vi "rename tag in mappings helper.vi"(8 "new tag name":string, 9 "input channel?":bool, 10 "old tag name":string, 11 "Mappings":T1[](array[typedef])) -> (3 "Mappings out":T1[](array[typedef]))   [LabVIEW 2013, in "engine configuration.lvclass"]
uses:
  engine configuration.lvclass
  <vilib>/NI/Tag Bus/table/mapping specification.ctl
  <vilib>/NI/Tag Bus/tag/Data Type.ctl
  <vilib>/NI/Tag Bus/table/mapping.ctl
  <vilib>/NI/Tag Bus/tag/tag descriptor.lvclass
  <vilib>/NI/Tag Bus/table/data table.lvlib
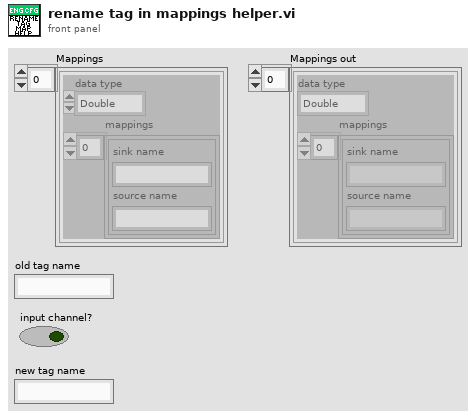
[diagram p1: front panel]
types:
  T1 = typedef "tag bus.lvlib/data table.lvlib/mapping specification.ctl" = cluster{"data type":T2, "mappings":T3[]}
  T2 = typedef "tag bus.lvlib/tag descriptor.lvclass/Data Type.ctl" = enum16{"Double", "Single", "I64", "I32", "I16", "I8", "U64", "U32", "U16", "U8", "Boolean", "String", "Array of Double", "Array of Single", "Array of I64", "Array of I32", "Array of I16", "Array of I8", "Array of U64", "Array of U32", "Array of U16", "Array of U8", "Array of Boolean", "Array of String"}
  T3 = typedef "tag bus.lvlib/data table.lvlib/mapping.ctl" = cluster{"sink name":string, "source name":string}
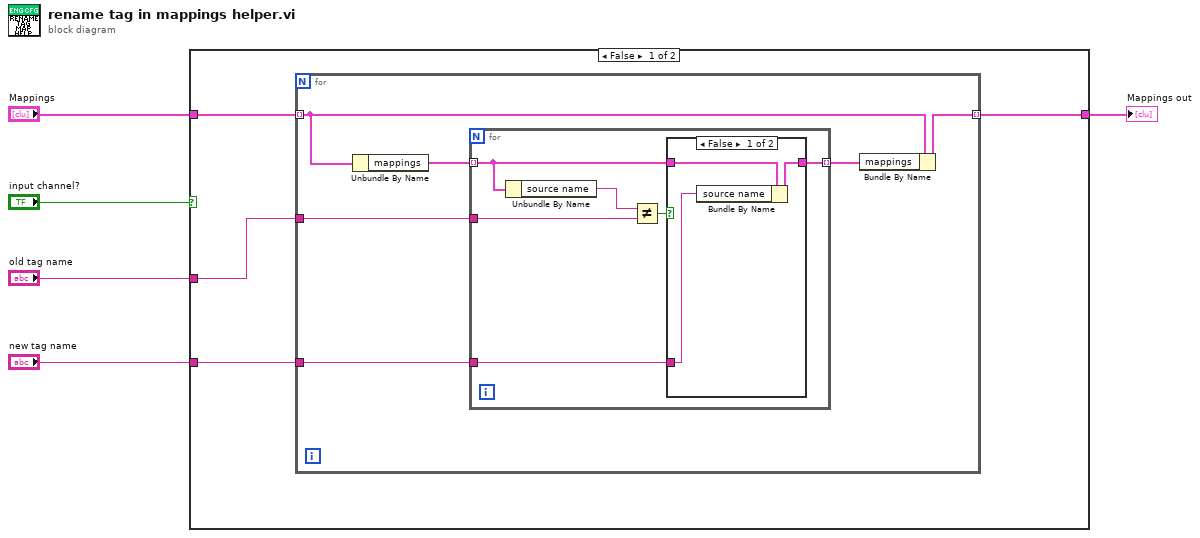
[diagram p0: block diagram]
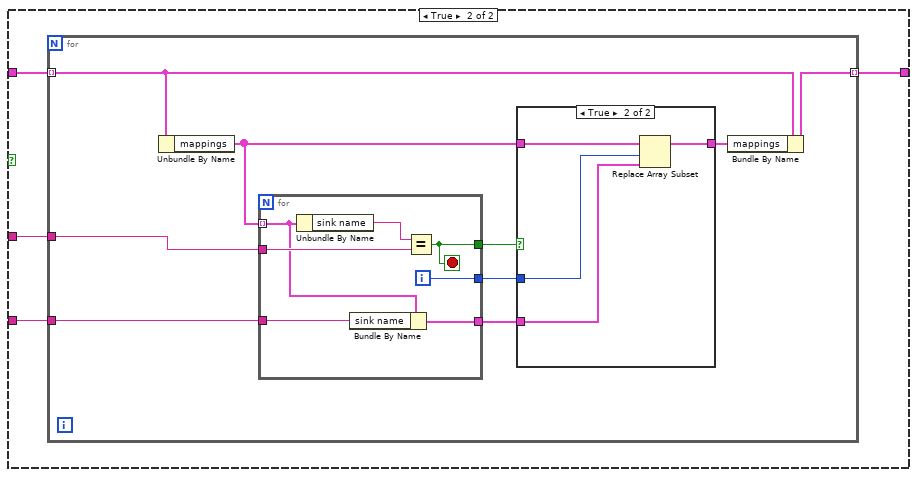
[diagram p3: hidden frame]
diagram:
  n1 = case shown="False" "input channel?" {
    tunnel: "Mappings" -> [w9 w29]
    tunnel: "old tag name" -> [w8 w28]
    tunnel: [w7 w27] -> w2
    tunnel: "new tag name" -> [w6 w26]
    frame False {
      n2 = for {
        tunnel: w9 -> [w13] mode=indexing
        tunnel: w8 -> [w14]
        tunnel: [w11] -> w7 mode=indexing
        tunnel: w6 -> [w10]
        n3 = Unbundle By Name(w13) -> ("mappings"=w15:T3[])
        n4 = for {
          tunnel: w15 -> [w18] mode=indexing
          tunnel: w14 -> [w20]
          tunnel: [w17] -> w12 mode=indexing
          tunnel: w10 -> [w16]
          n5 = Unbundle By Name(w18) -> ("source name"=w21:string)
          n6 = Not Equal?(x=w21, y=w20) -> (x != y?=w19:bool)
          n7 = case shown="False" w19 {
            tunnel: w18 -> [w24 w25]
            tunnel: [w22 w25] -> w17
            tunnel: w16 -> [w23 _]
            frame False {
              n8 = Bundle By Name(cluster=w24, "source name"=w23) -> (w22:T3)
            }
            frame True {
            }
          }
        }
        n9 = Bundle By Name(cluster=w13, "mappings"=w12) -> (w11:T1)
      }
    }
    frame True {
      n10 = for {
        tunnel: w29 -> [w38] mode=indexing
        tunnel: [w37] -> w27 mode=indexing
        tunnel: w28 -> [w36]
        tunnel: w26 -> [w31]
        n11 = Unbundle By Name(w38) -> ("mappings"=w34:T3[])
        n12 = for {
          tunnel: w34 -> [w46] mode=indexing
          tunnel: w36 -> [w49]
          tunnel: [w48] -> w32
          tunnel: [w47] -> w35
          tunnel: w31 -> [w45]
          tunnel: [w44] -> w30
          i -> [w48]
          stop <- w47 stop-if-true
          n13 = Unbundle By Name(w46) -> ("sink name"=w50:string)
          n14 = Bundle By Name(cluster=w46, "sink name"=w45) -> (w44:T3)
          n15 = Equal?(x=w50, y=w49) -> (x = y?=w47:bool)
        }
        n16 = case shown="True" w35 {
          tunnel: w34 -> [w39 w43]
          tunnel: [w39 w42] -> w33
          tunnel: w32 -> [_ w41]
          tunnel: w30 -> [_ w40]
          frame False {
          }
          frame True {
            n17 = Replace Array Subset(array=w43, new element=w40, index=w41) -> (w42:T3[])
          }
        }
        n18 = Bundle By Name(cluster=w38, "mappings"=w33) -> (w37:T1)
      }
    }
  }
  "Mappings out" <- w2
